vi "模块运行周期接口.vi"(11 "运行周期":T1={"运行模式"=enum."维护模式", "质控频次"=enum."关闭", "空白核查时间"=2, "跨度核查时间"=6, "测量间隔"=240} {"跨度核查时间" items=["00H", "01H", "02H", "03H", "04H", "05H", "06H", "07H", "08H", "09H", "10H", "11H", "12H", "13H", "14H", "15H", "16H", "17H", "18H", "19H", "20H", "21H", "22H", "23H", "关闭"]; "空白核查时间" items=["00H", "01H", "02H", "03H", "04H", "05H", "06H", "07H", "08H", "09H", "10H", "11H", "12H", "13H", "14H", "15H", "16H", "17H", "18H", "19H", "20H", "21H", "22H", "23H", "关闭"]}) -> ()   [LabVIEW 2016]
panel:
  # "运行模式："
  # "质控频次："
  # "零点核查时间："
  # "跨度核查时间："
  # "测量间隔："
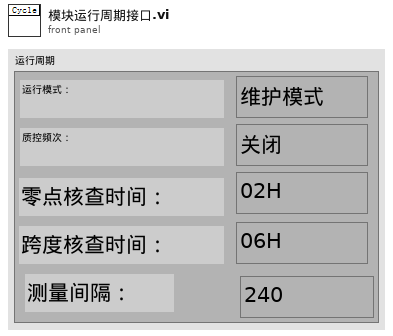
[diagram p1: front panel]
types:
  T1 = cluster{"运行模式":enum16{"维护模式", "常规模式", "应急模式", "质控模式"}, "质控频次":enum16{"关闭", "每天", "星期一", "星期二", "星期三", "星期四", "星期五", "星期六", "星期日"}, "空白核查时间":u16, "跨度核查时间":u16, "测量间隔":u16}
  T2 = cluster{"氨氮运行周期":cluster{"运行模式":enum16{"维护模式", "常规模式", "应急模式", "质控模式"}, "质控频次":enum16{"关闭", "每天", "星期一", "星期二", "星期三", "星期四", "星期五", "星期六", "星期日"}, "空白核查时间":u16, "跨度核查时间":u16, "测量间隔":u16}, "总磷运行周期":cluster{"运行模式":enum16{"维护模式", "常规模式", "应急模式", "质控模式"}, "质控频次":enum16{"关闭", "每天", "星期一", "星期二", "星期三", "星期四", "星期五", "星期六", "星期日"}, "空白核查时间":u16, "跨度核查时间":u16, "测量间隔":u16}, "总氮运行周期":cluster{"运行模式":enum16{"维护模式", "常规模式", "应急模式", "质控模式"}, "质控频次":enum16{"关闭", "每天", "星期一", "星期二", "星期三", "星期四", "星期五", "星期六", "星期日"}, "空白核查时间":u16, "跨度核查时间":u16, "测量间隔":u16}, "CODcr运行周期":cluster{"运行模式":enum16{"维护模式", "常规模式", "应急模式", "质控模式"}, "质控频次":enum16{"关闭", "每天", "星期一", "星期二", "星期三", "星期四", "星期五", "星期六", "星期日"}, "空白核查时间":u16, "跨度核查时间":u16, "测量间隔":u16}, "CODMn运行周期":cluster{"运行模式":enum16{"维护模式", "常规模式", "应急模式", "质控模式"}, "质控频次":enum16{"关闭", "每天", "星期一", "星期二", "星期三", "星期四", "星期五", "星期六", "星期日"}, "空白核查时间":u16, "跨度核查时间":u16, "测量间隔":u16}, "多参数运行周期":cluster{"运行模式":enum16{"维护模式", "常规模式", "应急模式", "质控模式"}, "质控频次":enum16{"关闭", "每天", "星期一", "星期二", "星期三", "星期四", "星期五", "星期六", "星期日"}, "空白核查时间":u16, "跨度核查时间":u16, "测量间隔":u16}}
  T3 = cluster{"运行模式":enum16{"维护模式", "常规模式", "应急模式", "质控模式"}, "24H周期设置":bool[]}
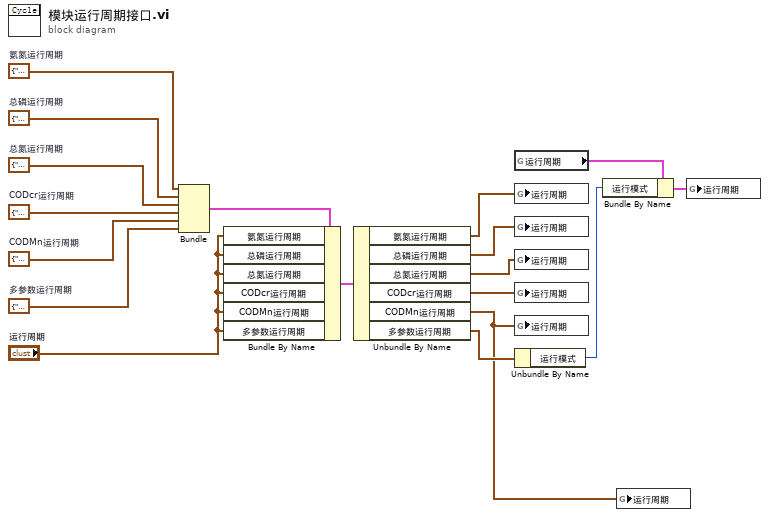
[diagram p0: block diagram]
diagram:
  w12 = T1 {"运行模式"=enum."维护模式", "质控频次"=enum."关闭", "空白核查时间"=2, "跨度核查时间"=6, "测量间隔"=4}  # 多参数运行周期
  w13 = T1 {"运行模式"=enum."维护模式", "质控频次"=enum."关闭", "空白核查时间"=2, "跨度核查时间"=6, "测量间隔"=4}  # CODMn运行周期
  w14 = T1 {"运行模式"=enum."维护模式", "质控频次"=enum."关闭", "空白核查时间"=2, "跨度核查时间"=6, "测量间隔"=4}  # CODcr运行周期
  w15 = T1 {"运行模式"=enum."维护模式", "质控频次"=enum."关闭", "空白核查时间"=2, "跨度核查时间"=6, "测量间隔"=4}  # 总氮运行周期
  w16 = T1 {"运行模式"=enum."维护模式", "质控频次"=enum."关闭", "空白核查时间"=2, "跨度核查时间"=6, "测量间隔"=4}  # 总磷运行周期
  w18 = T1 {"运行模式"=enum."维护模式", "质控频次"=enum."关闭", "空白核查时间"=2, "跨度核查时间"=6, "测量间隔"=4}  # 氨氮运行周期
  n1 = Bundle("氨氮运行周期"=w18, "总磷运行周期"=w16, "总氮运行周期"=w15, "CODcr运行周期"=w14, "CODMn运行周期"=w13, "多参数运行周期"=w12) -> (w17:T2)  [unwired: 1 in]
  n2 = Bundle By Name(cluster=w17, "氨氮运行周期"="运行周期", "总磷运行周期"="运行周期", "总氮运行周期"="运行周期", "CODcr运行周期"="运行周期", "CODMn运行周期"="运行周期", "多参数运行周期"="运行周期") -> (w10:T2)
  n3 = Unbundle By Name(w10) -> ("氨氮运行周期"=w9:T1, "总磷运行周期"=w4:T1, "总氮运行周期"=w3:T1, "CODcr运行周期"=w2:T1, "CODMn运行周期"=w1:T1, "多参数运行周期"=w6:T1)
  n4 = global read "断电保存变量.vi" "运行周期"() -> (w8:T3)
  n5 = global write "总磷总氮断电保存全局变量.vi" "运行周期"(w9) -> ()
  n6 = global write "总磷总氮断电保存全局变量.vi" "运行周期"(w4) -> ()
  n7 = global write "总磷总氮断电保存全局变量.vi" "运行周期"(w3) -> ()
  n8 = global write "总磷总氮断电保存全局变量.vi" "运行周期"(w2) -> ()
  n9 = global write "CODMn断电保存全局变量.vi" "运行周期"(w1) -> ()
  n10 = Unbundle By Name(w6) -> ("运行模式"=w5:enum16{"维护模式", "常规模式", "应急模式", "质控模式"})
  n11 = Bundle By Name(cluster=w8, "运行模式"=w5) -> (w7:T3)
  n12 = global write "CODMn断电保存全局变量.vi" "运行周期"(w1) -> ()
  n13 = global write "断电保存变量.vi" "运行周期"(w7) -> ()
